vi "Moving Average.vi"() -> ()   [LabVIEW 2019]
panel:
  out "Moving Average":dbl
  out "Current Value":dbl
  in  "stop":bool
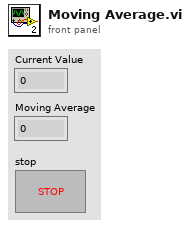
[diagram p1: front panel]
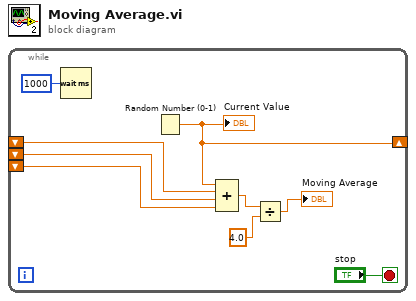
[diagram p0: block diagram]
diagram:
  n1 = while {
    shift-right: [w7] -> _
    shift-left: _ -> [w6]
    shift-left: _ -> [w5]
    shift-left: _ -> [w4]
    stop <- "stop" stop-if-true
    n2 = Wait (ms)(milliseconds to wait=u32 1000) -> ()  [unwired: 1 out]
    n3 = Random Number (0-1)() -> (number: 0 to 1=w7:dbl)
    "Current Value" <- w7
    n4 = Compound Arithmetic op=ADD(w7, w6, w5, w4) -> (w3:dbl)
    n5 = Divide(x=w3, y=4.0) -> (x/y=→"Moving Average":dbl)
  }
